vi "位移测试.vi"(15 "stop":bool) -> ()   [LabVIEW 2010]
uses:
  Instance           1 16Saved   位移测试 .vi
  Instance           2 16Saved   位移测试 .vi
  <vilib>/Utility/file.llb/Write To Spreadsheet File (DBL).vi
  <vilib>/Utility/file.llb/Read From Spreadsheet File (DBL).vi
  <vilib>/Analysis/NI_AALBase.lvlib
  <vilib>/Analysis/NI_AALPro.lvlib
panel:
  in  "比例系数":dbl=40.0 format="%.1f"
  in  "复位":bool
  out "灵敏度":dbl format="%.2f"
  in  "前进  回程":bool
  out "进回最大偏差":dbl format="%.2f"
  out "回程误差（%）":dbl format="%.2f"
  out "XY Graph 2":cluster{"all rows":dbl[], "all rows":dbl[]}[](graph)
  out "最大偏差":dbl format="%.2f"
  out "线性误差（%）":dbl format="%.2f"
  in  "显示测试结果":bool
  in  "记  数":bool
  in  "输入（x）":dbl format="%.1f"
  out "XY Graph":T1(graph)
  in  "实验人姓名":string
  out "输入信号（V）":dbl format="%.3f"
  out "当前位移（mm）":dbl format="%.3f"
  out "位移显示":dbl(graph) caption="位\n\n移"
  # "位移测试与系统静态特性实验"
  # "线\n性\n度"
  # "滞\n后\n度"
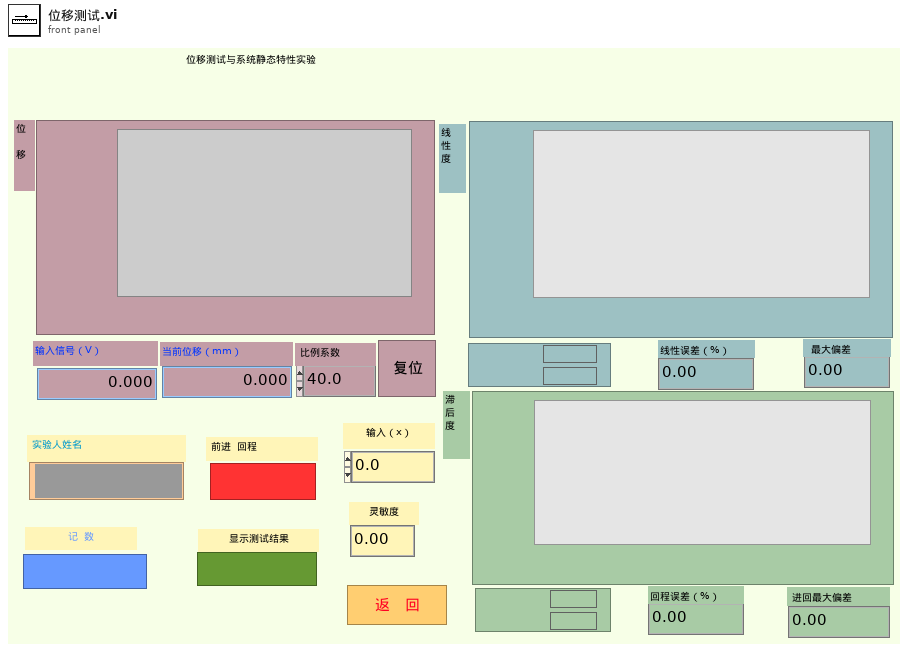
[diagram p1: front panel]
types:
  T1 = cluster{"all rows":dbl[], "Best Linear Fit":dbl[]}[]
  T2 = cluster{"all rows":dbl[], "Best Linear Fit":dbl[]}
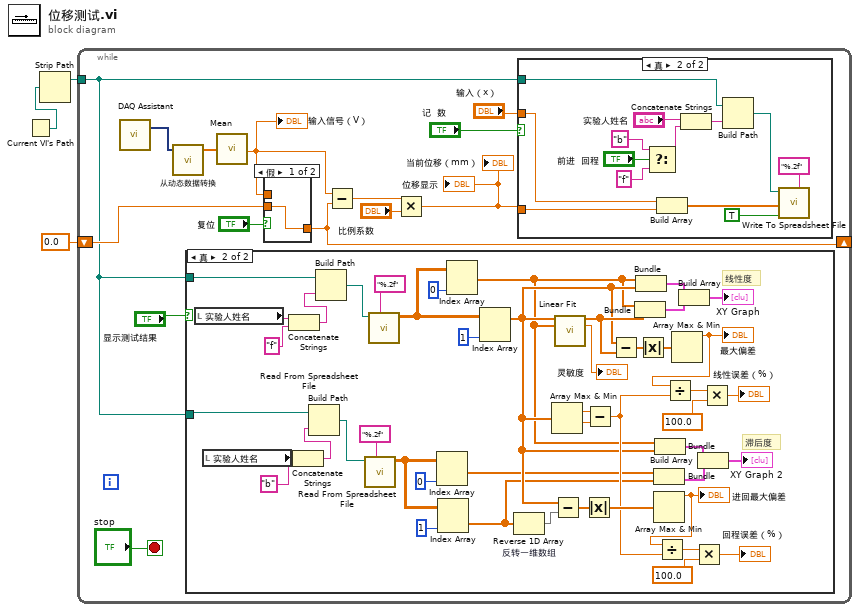
[diagram p0: block diagram]
diagram:
  n1 = Current VI's Path() -> (path=w2:path)
  n2 = Strip Path(path=w2) -> (stripped path=w1:path)  [unwired: 1 out]
  n3 = while {
    shift-left: 0.0 -> [w12]
    shift-right: [w11] -> _
    tunnel: w1 -> [w4]
    stop <- "stop" stop-if-true
    n4 = call "DAQ Assistant"() -> ("data"=w6:dynamicdata)  [unwired: 17 in, 2 out]
    n5 = call "从动态数据转换"("Dynamic Data Type"=w6) -> ("Array"=w5:dbl[])  [unwired: 3 in]
    n6 = case shown="真" "显示测试结果" {
      tunnel: w4 -> [_ w24]
      tunnel: w4 -> [_ w22]
      frame False {
      }
      frame True {
        # "滞后度"
        # "线性度"
        n7 = local read "实验人姓名"() -> (w49:string)
        n8 = local read "实验人姓名"() -> (w35:string)
        n9 = Concatenate Strings(w49, "f") -> (w21:string)
        n10 = Concatenate Strings(w35, "b") -> (w23:string)
        n11 = Build Path(base path=w24, name or relative path=w23) -> (appended path=w25:path)
        n12 = Build Path(base path=w22, name or relative path=w21) -> (appended path=w20:path)
        n13 = call-poly <vilib>:"Read From Spreadsheet File.vi"("format (%.3f)"="%.2f", "file path (dialog if empty)"=w25) -> ("all rows"=w37:dbl[][])  [unwired: 5 in, 4 out]
        n14 = call-poly <vilib>:"Read From Spreadsheet File.vi"("format (%.3f)"="%.2f", "file path (dialog if empty)"=w20) -> ("all rows"=w51:dbl[][])  [unwired: 5 in, 4 out]
        n15 = Index Array(array=w37, index (col)=0 ("Disabled Index")) -> (element=w29:dbl[])  [unwired: 1 in]
        n16 = Index Array(array=w37, index (col)=1 ("Disabled Index")) -> (element=w28:dbl[])  [unwired: 1 in]
        n17 = Index Array(array=w51, index (col)=0 ("Disabled Index")) -> (element=w30:dbl[])  [unwired: 1 in]
        n18 = Index Array(array=w51, index (col)=1 ("Disabled Index")) -> (element=w31:dbl[])  [unwired: 1 in]
        n19 = Reverse 1D Array "反转一维数组"(array=w28) -> (reversed array=w26:dbl[])
        n20 = Array Max & Min(array=w31) -> (max value=w56:dbl, min value=w55:dbl)  [unwired: 2 out]
        n21 = Subtract(x=w31, y=w26) -> (x-y=w45:dbl[])
        n22 = call <vilib>:"Linear Fit.vi"("Y"=w31, "X"=w30) -> ("Best Linear Fit"=w61:dbl[], "slope"=→"灵敏度":dbl)  [unwired: 9 in, 3 out]
        n23 = Absolute Value(x=w45) -> (abs(x)=w44:dbl[])
        n24 = Subtract(x=w56, y=w55) -> (x-y=w41:dbl)
        n25 = Subtract(x=w31, y=w61) -> (x-y=w60:dbl[])
        n26 = Bundle("all rows"=w30, "Best Linear Fit"=w61) -> (w62:T2)  [unwired: 1 in]
        n27 = Bundle("all rows"=w30, "all rows"=w31) -> (w63:cluster{"all rows":dbl[], "all rows":dbl[]})  [unwired: 1 in]
        n28 = Absolute Value(x=w60) -> (abs(x)=w59:dbl[])
        n29 = Bundle("all rows"=w29, "all rows"=w28) -> (w27:cluster{"all rows":dbl[], "all rows":dbl[]})  [unwired: 1 in]
        n30 = Array Max & Min(array=w44) -> (max value=w43:dbl)  [unwired: 3 out]
        "进回最大偏差" <- w43
        n31 = Bundle("all rows"=w30, "all rows"=w31) -> (w46:cluster{"all rows":dbl[], "all rows":dbl[]})  [unwired: 1 in]
        n32 = Divide(x=w43, y=w41) -> (x/y=w42:dbl)
        n33 = Array Max & Min(array=w59) -> (max value=w58:dbl)  [unwired: 3 out]
        "最大偏差" <- w58
        n34 = Divide(x=w58, y=w41) -> (x/y=w57:dbl)
        n35 = Build Array(w63, w62) -> (→"XY Graph":T1)
        n36 = Multiply(x=w42, y=100.0) -> (x*y=→"回程误差（%）":dbl)
        n37 = Build Array(w46, w27) -> (→"XY Graph 2":cluster{"all rows":dbl[], "all rows":dbl[]}[])
        n38 = Multiply(x=w57, y=100.0) -> (x*y=→"线性误差（%）":dbl)
      }
    }
    n39 = call <vilib>:"Mean.vi"("X"=w5) -> ("mean"=w8:dbl)  [unwired: 1 out]
    "输入信号（V）" <- w8
    n40 = case shown="假" "复位" {
      tunnel: w8 -> [_ w19]
      tunnel: [w18 w19] -> w11
      tunnel: w12 -> [w18 _]
      frame False {
      }
      frame True {
      }
    }
    n41 = Subtract(x=w8, y=w11) -> (x-y=w17:dbl)
    n42 = Multiply(x=w17, y="比例系数") -> (x*y=w9:dbl)
    "位移显示" <- w9
    "当前位移（mm）" <- w9
    n43 = case shown="真" "记  数" {
      tunnel: w9 -> [_ w78]
      tunnel: "输入（x）" -> [_ w70]
      tunnel: w4 -> [_ w69]
      frame False {
      }
      frame True {
        n44 = Select(t="b", s="前进  回程", f="f") -> (s? t:f=w71:string)
        n45 = Build Array(w70, w78) -> (w75:dbl[])
        n46 = Concatenate Strings("实验人姓名", w71) -> (w68:string)
        n47 = Build Path(base path=w69, name or relative path=w68) -> (appended path=w67:path)
        n48 = call-poly <vilib>:"Write To Spreadsheet File.vi"("format (%.3f)"="%.2f", "append to file? (new file:F)"=TRUE, "1D data"=w75, "file path (dialog if empty)"=w67) -> ()  [unwired: 4 in, 1 out]
      }
    }
  }
